vi "Read log file.vi"(0 "file path (use dialog)":path, 11 "error in":errorcluster) -> (4 "Array":T1[](array[typedef]), 15 "error out":errorcluster)   [LabVIEW 2012]
doc: "This Function is designed to read in a text file and retunr an array of string with each line of the text file. \n\nFor comments or questions about this code please look at the community example page below.\nhttp://decibel.ni.com/content/docs/DOC-10662"
uses:
  typedef/Log_User_Data.ctl
  typedef/User Accounts.ctl
panel:
  in  "Array 2":T1[](array[typedef])
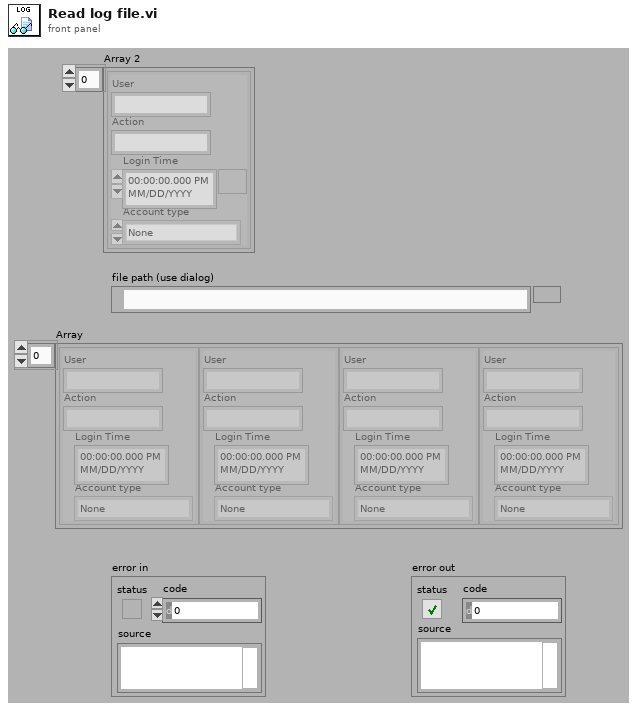
[diagram p1: front panel]
types:
  T1 = typedef "Log_User_Data.ctl" = cluster{"User":string, "Action":string, "Account type":T2, "Login Time ":timestamp}
  T2 = typedef "User Accounts.ctl" = enum16{"None", "User", "Admin"}
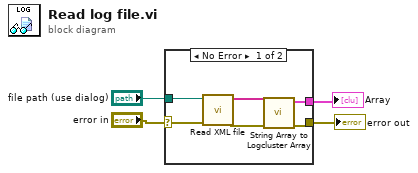
[diagram p0: block diagram]
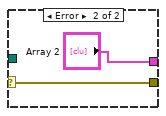
[diagram p2: hidden frame]
diagram:
  n1 = case shown="No Error" "error in" {
    selector: "error in" -> [w9 w12]
    tunnel: "file path (use dialog)" -> [w10 _]
    tunnel: [w6 w12] -> w3
    tunnel: [w7 "Array 2"] -> w1
    frame No Error {
      n2 = call "Read XML file.vi"("error in (no error)"=w9, "file path (use dialog)"=w10) -> ("error out"=w5:errorcluster, "Array 3"=w8:string[])  [unwired: 8 in]
      n3 = call "String Array to Logcluster Array.vi"("error in (no error)"=w5, "LogString Array"=w8) -> ("error out"=w6:errorcluster, "Array"=w7:T1[])  [unwired: 8 in]
    }
    frame Error {
    }
  }
  "error out" <- w3
  "Array" <- w1
